vi "BillardBorder.vi"(8 "error in (no error)":errorcluster, 10 "Dark Blue frame":T1={"Rmin"=0, "Gmin"=0, "Bmin"=121, "Rmax"=14, "Gmax"=42, "Bmax"=126}, 11 "path to PNG file":path) -> (0 "error out":errorcluster, 3 "Bords du billard":T2)   [LabVIEW 2019]
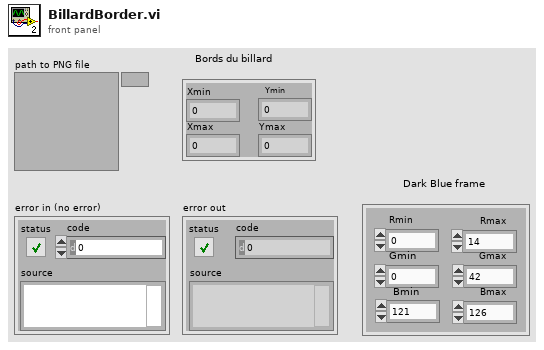
[diagram p1: front panel]
types:
  T1 = cluster{"Rmin":u32, "Gmin":u32, "Bmin":u32, "Rmax":u32, "Gmax":u32, "Bmax":u32}
  T2 = cluster{"Xmin":i32, "Ymin":i32, "Xmax":i32, "Ymax":i32}
  T3 = typedef "imagedata.ctl" = cluster{"image type":i32, "image depth":i32, "image":u8[], "mask":u8[], "colors":u32[], "Rectangle":cluster{"left":i16, "top":i16, "right":i16, "bottom":i16}}
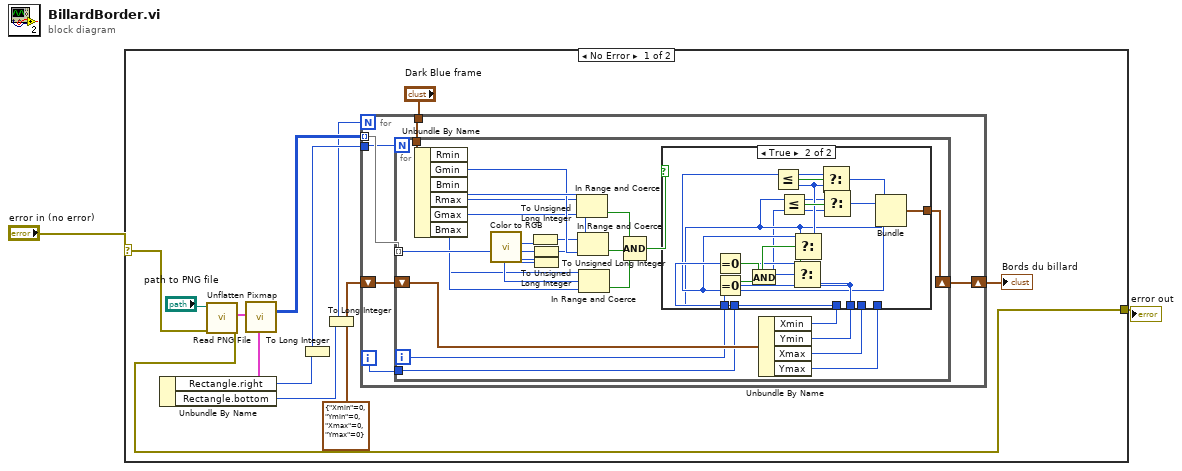
[diagram p0: block diagram]
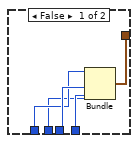
[diagram p2: hidden frame]
diagram:
  n1 = case shown="No Error" "error in (no error)" {
    selector: "error in (no error)" -> [w4 w66]
    tunnel: [w3 w66] -> w1
    frame No Error {
      n2 = call <vilib>:"Read PNG File.vi"("error in (no error)"=w4, "path to PNG file"="path to PNG file") -> ("error out"=w3:errorcluster, "image data"=w9:T3)  [unwired: 7 in, 1 out]
      n3 = Unbundle By Name(w9) -> ("Rectangle.right"=w8:i16, "Rectangle.bottom"=w6:i16)
      n4 = call <vilib>:"Unflatten Pixmap.vi"("image data"=w9) -> ("24-bit pixmap"=w13:u32[][])  [unwired: 4 in, 6 out]
      n5 = To Long Integer(number=w8) -> (32bit integer=w7:i32)
      n6 = To Long Integer(number=w6) -> (32bit integer=w5:i32)
      n7 = for {
        N: w5 -> [_]
        tunnel: w13 -> [w20] mode=indexing
        tunnel: "Dark Blue frame" -> [w19]
        shift-right: [w18] -> w10
        shift-left: T2 {"Xmin"=0, "Ymin"=0, "Xmax"=0, "Ymax"=0} -> [w17]
        tunnel: w7 -> [w15]
        i -> [w16]
        n8 = for {
          N: w15 -> [_]
          tunnel: w20 -> [w46] mode=indexing
          tunnel: w19 -> [w42]
          shift-right: [w27] -> w18
          shift-left: w17 -> [w29]
          tunnel: w16 -> [w26]
          i -> [w28]
          n9 = Unbundle By Name(w42) -> ("Rmin"=w41:u32, "Gmin"=w40:u32, "Bmin"=w33:u32, "Rmax"=w39:u32, "Gmax"=w38:u32, "Bmax"=w32:u32)
          n10 = call <vilib>:"Color to RGB.vi"("Color"=w46) -> ("R"=w36:u8, "G"=w31:u8, "B"=w35:u8)  [unwired: 1 out]
          n11 = To Unsigned Long Integer(number=w36) -> (unsigned 32bit integer=w37:u32)
          n12 = To Unsigned Long Integer(number=w31) -> (unsigned 32bit integer=w30:u32)
          n13 = To Unsigned Long Integer(number=w35) -> (unsigned 32bit integer=w34:u32)
          n14 = In Range and Coerce(upper limit=w39, x=w37, lower limit=w41) -> (In Range?=w45:bool)  [unwired: 1 out]
          n15 = In Range and Coerce(upper limit=w38, x=w30, lower limit=w40) -> (In Range?=w44:bool)  [unwired: 1 out]
          n16 = In Range and Coerce(upper limit=w32, x=w34, lower limit=w33) -> (In Range?=w43:bool)  [unwired: 1 out]
          n17 = Compound Arithmetic op=AND(w45, w44, w43) -> (w21:bool)
          n18 = Unbundle By Name(w29) -> ("Xmin"=w23:i32, "Ymin"=w22:i32, "Xmax"=w25:i32, "Ymax"=w24:i32)
          n19 = case shown="True" w21 {
            tunnel: w25 -> [w49 _]
            tunnel: w28 -> [_ w57]
            tunnel: [w51 w65] -> w27
            tunnel: w24 -> [w50 _]
            tunnel: w26 -> [_ w55]
            tunnel: w23 -> [w48 w61]
            tunnel: w22 -> [w47 w60]
            frame False {
              n20 = Bundle("Xmin"=w48, "Ymin"=w47, "Xmax"=w49, "Ymax"=w50) -> (w51:T2)  [unwired: 1 in]
            }
            frame True {
              n21 = Equal To 0?(x=w61) -> (x = 0?=w63:bool)
              n22 = Equal To 0?(x=w60) -> (x = 0?=w64:bool)
              n23 = And(x=w63, y=w64) -> (x .and. y?=w62:bool)
              n24 = Select(t=w55, s=w62, f=w60) -> (s? t:f=w54:i32)
              n25 = Less Or Equal?(x=w55, y=w54) -> (x <= y?=w59:bool)
              n26 = Select(t=w57, s=w62, f=w61) -> (s? t:f=w56:i32)
              n27 = Less Or Equal?(x=w57, y=w56) -> (x <= y?=w58:bool)
              n28 = Select(t=w57, s=w58, f=w56) -> (s? t:f=w52:i32)
              n29 = Select(t=w55, s=w59, f=w54) -> (s? t:f=w53:i32)
              n30 = Bundle("Xmin"=w52, "Ymin"=w53, w57, w55) -> (w65:cluster{"Xmin":i32, "Ymin":i32, i32, i32})  [unwired: 1 in]
            }
          }
        }
      }
      "Bords du billard" <- w10
    }
    frame Error {
    }
  }
  "error out" <- w1
